vi "getDetailedState.vi"(11 "Model in":refnum<class "Model.lvclass">) -> (2 "DetailedStates":T1=enum."StandbyState", 3 "Model out":refnum<class "Model.lvclass">)   [LabVIEW 2016, in "Model.lvclass"]
uses:
  Model.lvclass
  DataTypes/Topics/Parts/DetailedStates.ctl
  Model.lvclass/Model.ctl
  DataTypes/Topics/M1M3SupportTopics.lvlib
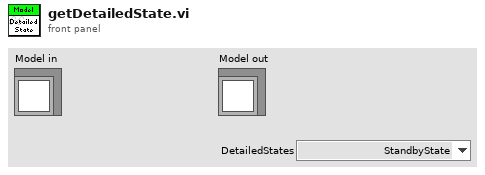
[diagram p1: front panel]
types:
  T1 = typedef "M1M3SupportTopics.lvlib/DetailedStates.ctl" = enum16{"OfflineState", "InitialState", "StandbyState", "DisabledState", "ParkedState", "FaultState", "ParkedMaintenanceState", "ActiveMaintenanceState"}
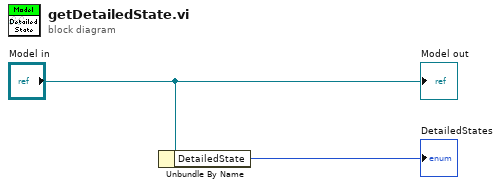
[diagram p0: block diagram]
diagram:
  n1 = Unbundle By Name("Model in") -> ("DetailedState"=→"DetailedStates":T1)
  "Model out" <- "Model in"
